vi "Meas Result Fill Freq Selector.vi"(2 "meas":T1={"swp cfg"={"N"=0, "R"=0, "f list"=[], "smpl delay"=0.0, "set delay"=0.0, "set delay np"=0.0, "meas root"=path "", "meas name"="", "meas a-index"=FALSE, "rnd sweep"=FALSE, "mode"=enum."Frequency", "swp mode"=enum."Linear", "avg"=0, "subrec"=0, "multi-freq"=FALSE, "selfcal"=FALSE, "selfcal period [h]"=0.0}, "bridge"={"type"=enum."TWM client", "TWM"={"pipe name"="", "parameters"=[], "handle"=0, "fixed aper [s]"=0.0, "f-list [Hz]"=[], "discrete f-list"=FALSE, "unc mode"=enum."None", "unc mcc"=0, "unc first"=FALSE, "alg id"=enum."TWM-LowZ - Low Z measurement"}, "last f"=0.0, "bias comp"={"bias type"=enum."dummy", "VISA"="", "Enable"=FALSE, "channel qu"=[], "channel Uinit"=[]}, "sim mode"=enum."Generic RLC network", "channel idns"=[], "sim phases"=1}, "src"={"type"=enum."Tektronix AFG3101C", "idn"="", "afg"={"VISA"="", "const"=0.0, "gen DC"=FALSE, "ext ref"=FALSE}, "cDAQ dds"={"device"="", "channels"=[], "mclk source"="", "mclk [Hz]"=0.0, "fs [Hz]"=0.0, "block [s]"=0.0, "buf [s]"=0.0, "task"="", "cmd queue"=refnum, "proc ref"=refnum, "smpl clock out"="/cDAQ3/PFI0", "export smpl clock"=FALSE, "DC ofs [V]"=[], "timebase source"="", "timebase mode"=enum."Local", "dither"=enum."Disabled", "dither level"=0.0, "phase [rad]"=[]}, "gain [V/A]"=1.0, "F5xxx session"={"VISA"="", "mode"=enum."AC voltage", "Earth on"=FALSE, "Ext ref lock"=FALSE}, "t3awg"={"VISA"="", "use ext ref"=FALSE, "ext ref [Hz]"=0.0, "load Z"=enum."High Z", "ramdac max n"=0, "noise dither [V]"=0.0, "t3awg fs rules"=[], "channels"=0, "ramdac min n"=0, "channel list"=[], "gen resl [Vpp]"=0.0, "wave data format"=enum."Binary"}}, "results"=refnum, "dvm"={"type"=enum."Disabled", "idn"="", "F5790"={"VISA"="", "Input"=enum."input 1", "Digital filter restart"=enum."medium", "hi resolution"=enum."off", "Digital filter mode"=enum."off", "ext guard"=FALSE}, "HP3458A"={"VISA"="", "ac method"=0, "resolution"=enum."6.5", "function"=0, "frequency source"=3, "auto range"=1, "manual range"=1.0}}, "thermo"={"type"=enum."COMET Tx5xx (ethernet)", "comment"="", "tag"="", "refresh"=5.0, "IP"="", "port"=502, "VISA"="", "last readout"=timestamp(0 s since 1904-01-01), "TCP ref"=refnum, "VISA sess"="", "idn"="", "press"=0.0, "RH"=0.0, "temp"=0.0, "pres cor"=[], "RH cor"=[], "temp cor"=[], "try left"=0, "failed"=FALSE, "RTD set"=[], "RTD inv"=[], "range"=0.0, "net mode"=enum."MODBUS", "try fail"=enum."Stop trying - return NaN", "timeout [s]"=0.0, "max retries"=0, "sim t [deg]"=0.0, "status"=0}} {"thermo"."status" items=["ok", "retry", "failed"]; "thermo"."RTD inv" format="%.1f"; "thermo"."RTD set" format="%.1f"; "thermo"."temp cor" format="%.1f"; "thermo"."RH cor" format="%.1f"; "thermo"."pres cor" format="%.1f"; "thermo"."refresh" min=0.1 max=1000.0 format="%.2f"; "dvm"."HP3458A"."manual range" format="%_3g"; "dvm"."HP3458A"."auto range" items=["OFF", "ON", "ONCE"]; "dvm"."HP3458A"."frequency source" items=["AC + DC Current", "AC + DC Voltage", "AC Current", "AC Voltage"]; "dvm"."HP3458A"."function" items=["DC Voltage", "AC Voltage", "AC + DC Voltage", "DC Current", "AC Current", "AC + DC Current", "2-Wire Resistance", "4-Wire Resistance", "Frequency", "Period", "Direct Sampling DC", "Direct Sampling AC", "Sub-Sampling DC", "Sub-Sampling AC"]; "dvm"."HP3458A"."ac method" items=["Analog", "Random", "Synchronous"]; "src"."t3awg"."t3awg fs rules"."fs-step [Hz]" format="%#_6p"; "src"."t3awg"."t3awg fs rules"."fs-max [Hz]" format="%#_6p"; "src"."t3awg"."t3awg fs rules"."for f0 <" format="%#_6p"; "src"."t3awg"."t3awg fs rules"."fs-min [Hz]" format="%#_6p"; "src"."cDAQ dds"."channels" min=0 step=1; "bridge"."TWM"."f-list [Hz]" format="%#_6p"; "swp cfg"."f list"."bias" format="%#_3p"; "swp cfg"."f list"."level" format="%#_3p"; "swp cfg"."f list"."fs [Hz]" format="%#_5p"; "swp cfg"."f list"."time [s]" format="%#_3p"; "swp cfg"."f list"."f/fs" format="%#_3p"; "swp cfg"."f list"."periods" format="%#_3f"; "swp cfg"."f list"."f [Hz]" format="%#_5p"}, 3 "results data":T36, 4 "res fid":refnum<vi>) -> (0 "freq filter (NaN: no filter)":dbl, 1 "freq index (default: 0)":u16)   [LabVIEW 2020]
doc: "Fills list of frequencies selector based on available sweep spots cout available in result data."
uses:
  Meas Results.ctl
  bridge/Bridge Frequency Readings Data.ctl
  drivers/TWM client/Meas Proc QWTB Spectrum Data.ctl
  drivers/TWM client/TWM Phase Info.ctl
  meas session.ctl
  Meas Sweep Config.ctl
  Meas Freq Info.ctl
  meas_swp_mode.ctl
  meas_sweep_flist_mode.ctl
  bridge/Bridge Session.ctl
  bridge/Bridge Type.ctl
  drivers/TWM client/TWM Session.ctl
  drivers/TWM client/TWM parameters.ctl
  drivers/TWM client/Meas Proc QWTB Uncertainty Mode.ctl
  bridge/Bridge Algorithm.ctl
  bridge/Bridge Bias Session.ctl
  bridge/Bridge Bias Type.ctl
  bridge/Bridge Sim Mode.ctl
  source/Source Session.ctl
  source/Source Type.ctl
  drivers/AFG3101C/AFG3101C Session.ctl
  drivers/cDAQ DDS/cDAQ DDS Session.ctl
  drivers/cDAQ DDS/cDAQ DDS Setup.ctl
  drivers/cDAQ DDS/cDAQ DDS Timebase Mode.ctl
  drivers/cDAQ DDS/cDAQ DDS Dither.ctl
  drivers/Fluke 5XXX/top_lev/F5xxx_session.ctl
  drivers/Fluke 5XXX/top_lev/F5xxx_output_mode.ctl
  drivers/T3AWG3K/toplevel/T3AWG Session.ctl
  drivers/T3AWG3K/toplevel/T3AWG Load Z.ctl
  drivers/T3AWG3K/toplevel/fgen_ramdac_fs_rules.ctl
  drivers/T3AWG3K/toplevel/T3AWG Channel.ctl
  Meas Results Ref.ctl
  dvm/dvm session.ctl
  dvm/dvm type.ctl
  drivers/Fluke 5790A/top_level/F5790 session.ctl
  drivers/Agilent 3458A/top level/HP3458A Session.ctl
  thermo/thermo.ctl
  thermo/thermo_types.ctl
  thermo/Thermometer Fail Action.ctl
  drivers/T3AWG3K/Active Technologies AWG3000.lvlib
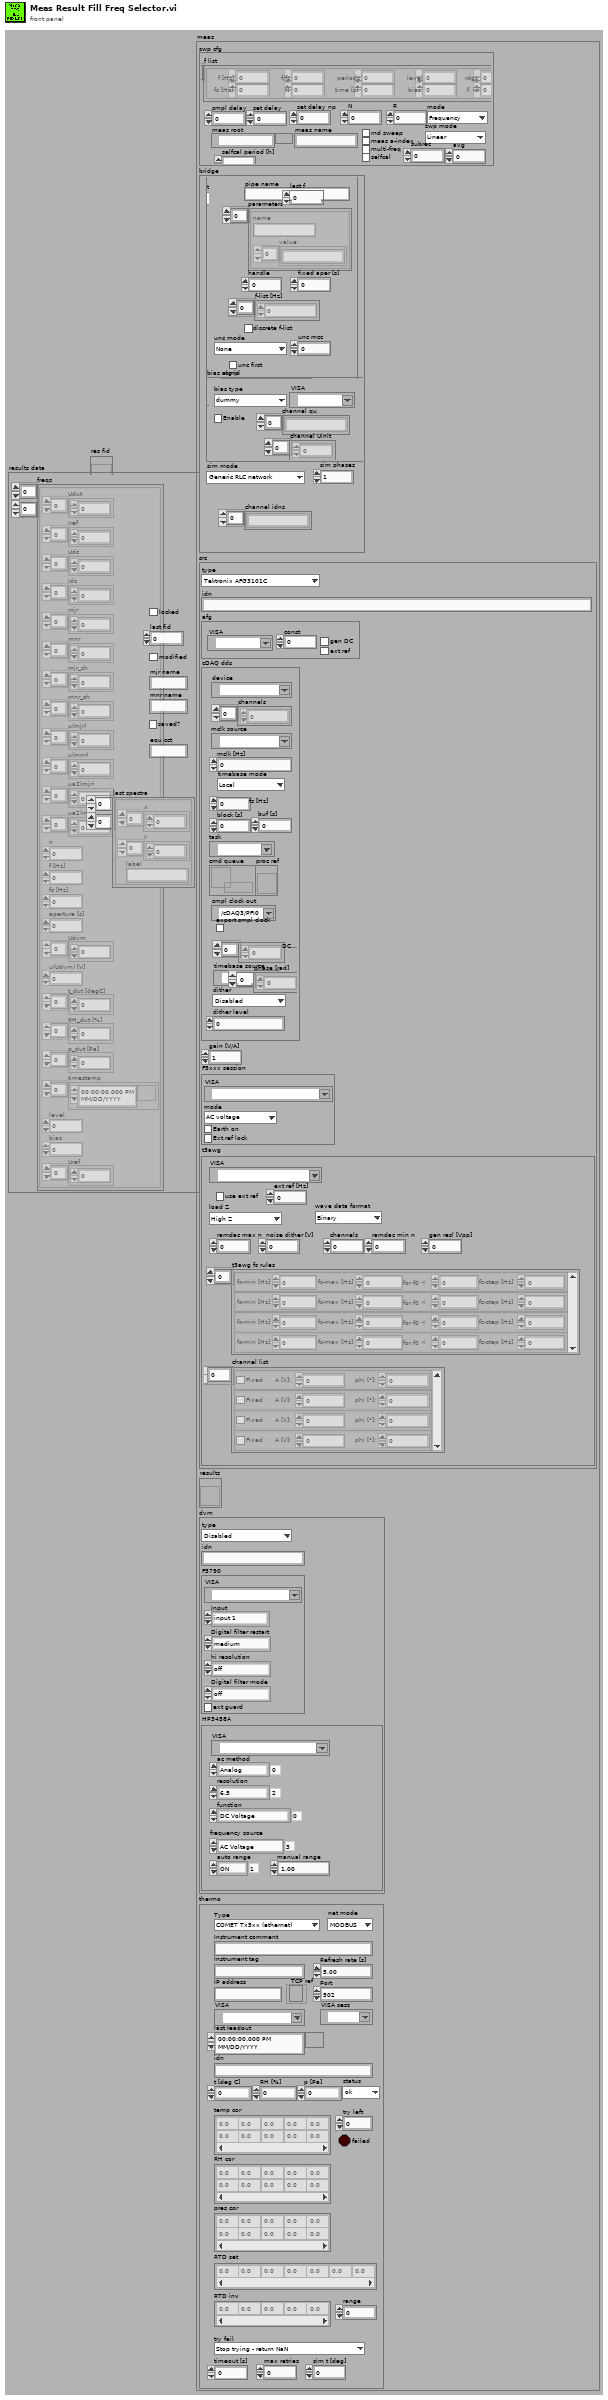
[diagram p1: front panel]
types:
  T1 = typedef "meas session.ctl" = cluster{"swp cfg":T2, "bridge":T6, "src":T15, "results":T28, "dvm":T29, "thermo":T33}
  T2 = typedef "Meas Sweep Config.ctl" = cluster{"N":i32, "R":i32, "f list":T3[], "smpl delay":dbl, "set delay":dbl, "set delay np":dbl, "meas root":path, "meas name":string, "meas a-index":bool, "rnd sweep":bool, "mode":T4, "swp mode":T5, "avg":i32, "subrec":i32, "multi-freq":bool, "selfcal":bool, "selfcal period [h]":dbl}
  T3 = typedef "Meas Freq Info.ctl" = cluster{"f [Hz]":dbl, "periods":dbl, "f/fs":dbl, "time [s]":dbl, "fs [Hz]":dbl, "N":i32, "level":dbl, "bias":dbl, "rdgs":i32, "f. id":i32}
  T4 = typedef "meas_swp_mode.ctl" = enum16{"Frequency", "Level", "Bias"}
  T5 = typedef "meas_sweep_flist_mode.ctl" = enum16{"Linear", "Log10"}
  T6 = typedef "Bridge Session.ctl" = cluster{"type":T7, "TWM":T8, "last f":dbl, "bias comp":T12, "sim mode":T14, "channel idns":string[], "sim phases":i32}
  T7 = typedef "Bridge Type.ctl" = enum16{"TWM client", "dummy"}
  T8 = typedef "TWM Session.ctl" = cluster{"pipe name":string, "parameters":T9[], "handle":i32, "fixed aper [s]":dbl, "f-list [Hz]":dbl[], "discrete f-list":bool, "unc mode":T10, "unc mcc":i32, "unc first":bool, "alg id":T11}
  T9 = typedef "TWM parameters.ctl" = cluster{"name":string, "value":string[]}
  T10 = typedef "Meas Proc QWTB Uncertainty Mode.ctl" = enum16{"None", "GUF", "Monte Carlo"}
  T11 = typedef "Bridge Algorithm.ctl" = enum16{"TWM-LowZ - Low Z measurement", "TWM-InpZ - Digitizer input Z measurement", "TWM-TIAZ - High Z using TIA"}
  T12 = typedef "Bridge Bias Session.ctl" = cluster{"bias type":T13, "VISA":refnum<visa-resource-name>, "Enable":bool, "channel qu":string[], "channel Uinit":dbl[]}
  T13 = typedef "Bridge Bias Type.ctl" = enum16{"dummy", "CMI LiBbias V1.0"}
  T14 = typedef "Bridge Sim Mode.ctl" = enum16{"Generic RLC network", "Interchannel transfer", "Input impedance"}
  T15 = typedef "Source Session.ctl" = cluster{"type":T16, "idn":string, "afg":T17, "cDAQ dds":T18, "gain [V/A]":dbl, "F5xxx session":T21, "t3awg":T23}
  T16 = typedef "Source Type.ctl" = enum16{"Tektronix AFG3101C", "cDAQ DAC", "Fluke 5xxx", "Datron 4xxx", "Agilent 33120A", "R&S SMT", "Teledyne LeCroy T3AWG", "dummy"}
  T17 = typedef "AFG3101C Session.ctl" = cluster{"VISA":refnum<visa-resource-name>, "const":dbl, "gen DC":bool, "ext ref":bool}
  T18 = typedef "cDAQ DDS Session.ctl" = cluster{"device":tag, "channels":i32[], "mclk source":tag, "mclk [Hz]":dbl, "fs [Hz]":dbl, "block [s]":dbl, "buf [s]":dbl, "task":refnum<k21>, "cmd queue":refnum<queue>, "proc ref":refnum<vi>, "smpl clock out":tag, "export smpl clock":bool, "DC ofs [V]":dbl[], "timebase source":tag, "timebase mode":T19, "dither":T20, "dither level":dbl, "phase [rad]":dbl[]}
  T19 = typedef "cDAQ DDS Timebase Mode.ctl" = enum16{"Local", "Take from ADC (e.g. NI 9238)", "Other source"}
  T20 = typedef "cDAQ DDS Dither.ctl" = enum16{"Disabled", "Gaussian"}
  T21 = typedef "F5xxx_session.ctl" = cluster{"VISA":refnum<visa-resource-name>, "mode":T22, "Earth on":bool, "Ext ref lock":bool}
  T22 = typedef "F5xxx_output_mode.ctl" = enum16{"AC voltage", "AC current"}
  T23 = typedef "Active Technologies AWG3000.lvlib/T3AWG Session.ctl" = cluster{"VISA":refnum<visa-resource-name>, "use ext ref":bool, "ext ref [Hz]":dbl, "load Z":T24, "ramdac max n":i32, "noise dither [V]":dbl, "t3awg fs rules":T25[], "channels":i32, "ramdac min n":i32, "channel list":T26[], "gen resl [Vpp]":dbl, "wave data format":T27}
  T24 = typedef "Active Technologies AWG3000.lvlib/T3AWG Load Z.ctl" = enum16{"High Z", "50 Ohm"}
  T25 = typedef "Active Technologies AWG3000.lvlib/fgen_ramdac_fs_rules.ctl" = cluster{"fs-min [Hz]":dbl, "fs-max [Hz]":dbl, "for f0 < ":dbl, "fs-step [Hz]":dbl}
  T26 = typedef "Active Technologies AWG3000.lvlib/T3AWG Channel.ctl" = cluster{"Fixed":bool, "A [V]:":dbl, "phi [°]:":dbl}
  T27 = typedef "Active Technologies AWG3000.lvlib/T3AWG Wave Format" = enum16{"Text", "Binary"}
  T28 = typedef "Meas Results Ref.ctl" = refnum<vi>
  T29 = typedef "dvm session.ctl" = cluster{"type":T30, "idn":string, "F5790":T31, "HP3458A":T32}
  T30 = typedef "dvm type.ctl" = enum16{"Disabled", "Simulated", "Fluke 5790A", "Keysight 3458A"}
  T31 = typedef "F5790 session.ctl" = cluster{"VISA":refnum<visa-resource-name>, "Input":enum16{"input 1", "input 2", "wide-band"}, "Digital filter restart":enum16{"medium", "fine", "coarse"}, "hi resolution":enum16{"off", "on"}, "Digital filter mode":enum16{"off", "fast", "medium", "slow"}, "ext guard":bool}
  T32 = typedef "HP3458A Session.ctl" = cluster{"VISA":refnum<visa-resource-name>, "ac method":u16, "resolution":enum16{"4.5", "5.5", "6.5", "7.5", "8.5"}, "function":u16, "frequency source":u16, "auto range":u16, "manual range":dbl}
  T33 = typedef "thermo.ctl" = cluster{"type":T34, "comment":string, "tag":string, "refresh":dbl, "IP":string, "port":u16, "VISA":refnum<visa-resource-name>, "last readout":timestamp, "TCP ref":refnum<k5>, "VISA sess":refnum<visa-resource-name>, "idn":string, "press":dbl, "RH":dbl, "temp":dbl, "pres cor":dbl[][], "RH cor":dbl[][], "temp cor":dbl[][], "try left":i32, "failed":bool, "RTD set":dbl[], "RTD inv":dbl[], "range":dbl, "net mode":enum16{"MODBUS", "HTTP"}, "try fail":T35, "timeout [s]":dbl, "max retries":i32, "sim t [deg]":dbl, "status":u16}
  T34 = typedef "thermo_types.ctl" = enum16{"Disabled", "Simulated", "COMET Tx5xx (ethernet)", "Keithley 2002 (GPIB) + RTD", "Agilent 344xx (GPIB) + RTD"}
  T35 = typedef "Thermometer Fail Action.ctl" = enum16{"Stop trying - keep last value", "Stop trying - return NaN", "Generate error - stop sweep"}
  T36 = typedef "Meas Results.ctl" = cluster{"freqs":T37[][], "locked":bool, "last fid":i32, "modified":bool, "mjr name":string, "mnr name":string, "last spectra":T38[][], "saved?":bool, "TWM phase":T39[], "time start":timestamp, "time stop":timestamp, "equ cct":string}
  T37 = typedef "Bridge Frequency Readings Data.ctl" = cluster{"Udut":dbl[], "Iref":dbl[], "Udc":dbl[], "Idc":dbl[], "mjr":dbl[], "mnr":dbl[], "mjr_sh":dbl[], "mnr_sh":dbl[], "u(mjr)":dbl[], "u(mnr)":dbl[], "ua2(mjr)":dbl[], "ua2(mnr)":dbl[], "n":i32, "f [Hz]":dbl, "fs [Hz]":dbl, "aperture [s]":dbl, "Udvm":dbl[], "u(Udvm) [V]":dbl, "t_dut [degC]":dbl[], "RH_dut [%]":dbl[], "p_dut [Pa]":dbl[], "timestamp":timestamp[], "level":dbl, "bias":dbl, "Uref":dbl[]}
  T38 = typedef "Meas Proc QWTB Spectrum Data.ctl" = cluster{"x":sgl[], "y":sgl[], "label":string}
  T39 = typedef "TWM Phase Info.ctl" = cluster{"ref chn id (I)":string, "dut chn id (U)":string, "ref chn range [V]":dbl, "dut chn range [V]":dbl, "aperture [s]":dbl, "fs [Hz]":dbl, "ref chn transducer (I)":string, "dut chn transducer (U)":string}
  T40 = enum8{"Enabled", "Disabled", "Disabled and Grayed Out"}
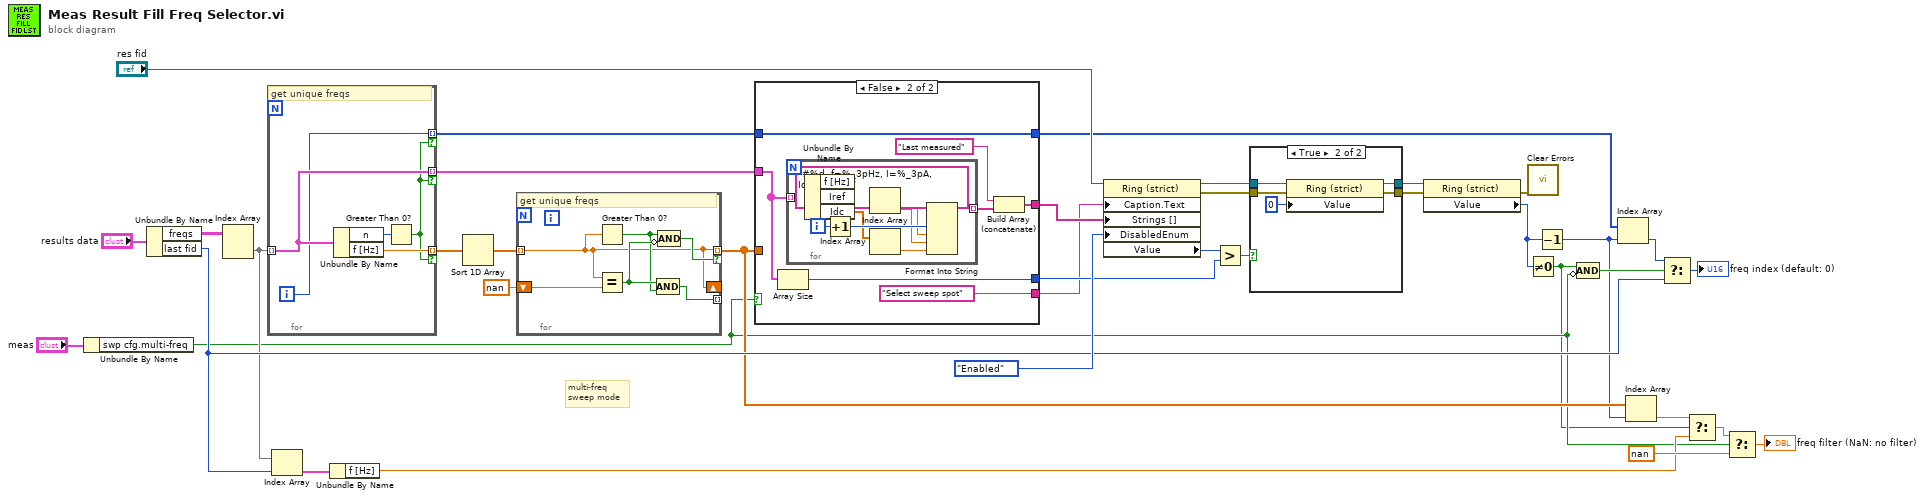
[diagram p0: block diagram]
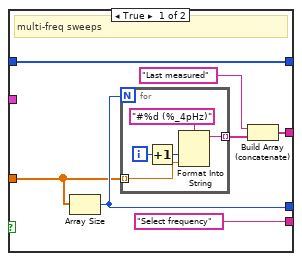
[diagram p2: hidden frame]
diagram:
  # "multi-freq\nsweep mode"
  n1 = Unbundle By Name("meas") -> ("swp cfg.multi-freq"=w10:bool)
  n2 = Unbundle By Name("results data") -> ("freqs"=w32:T37[][], "last fid"=w22:i32)
  n3 = Index Array(array=w32) -> (element=w20:T37[])  [unwired: 2 in]
  n4 = for {
    tunnel: w20 -> [w40] mode=indexing
    tunnel: [w42] -> w15 mode=indexing if=w38
    tunnel: [w40] -> w5 mode=indexing if=w38
    tunnel: [w39] -> w4 mode=indexing if=w38
    i -> [w39]
    # "get unique freqs"
    n5 = Unbundle By Name(w40) -> ("n"=w41:i32, "f [Hz]"=w42:dbl)
    n6 = Greater Than 0?(x=w41) -> (x > 0?=w38:bool)
  }
  n7 = Index Array(array=w20, index=w22) -> (element=w21:T37)
  n8 = Unbundle By Name(w21) -> ("f [Hz]"=w18:dbl)
  n9 = Sort 1D Array(array=w15) -> (sorted array=w12:dbl[])
  n10 = for {
    tunnel: w12 -> [w43] mode=indexing
    shift-right: [w43] -> _
    shift-left: nan ("f [Hz]") -> [w48]
    tunnel: [w44] -> _ mode=indexing
    tunnel: [w43] -> w13 mode=indexing if=w47
    # "get unique freqs"
    n11 = Greater Than 0?(x=w43) -> (x > 0?=w45:bool)
    n12 = Equal?(x=w43, y=w48) -> (x = y?=w46:bool)
    n13 = Compound Arithmetic op=AND(w46, w45) -> (w44:bool)
    n14 = Compound Arithmetic op=AND(w45, invert w46) -> (w47:bool)
  }
  n15 = case shown="False" w10 {
    tunnel: [w55 w67] -> w26
    tunnel: w13 -> [w54 _]
    tunnel: [w53 w66] -> w25
    tunnel: w5 -> [_ w61]
    tunnel: ["Select frequency" "Select sweep spot"] -> w17
    tunnel: w4 -> [w49 w62]
    tunnel: [w49 w62] -> w2
    frame True {
      # "multi-freq sweeps"
      n16 = Array Size(array=w54) -> (size(s)=w55:i32)
      n17 = for {
        N: w55 -> [_]
        tunnel: [w57] -> w52 mode=indexing
        tunnel: w54 -> [w56] mode=indexing
        i -> [w60]
        n18 = Increment(x=w60) -> (x+1=w59:i32)
        n19 = Format Into String(format string="#%d (%_4pHz)", w59, w56) -> (resulting string=w57:string)  [unwired: 2 in, 1 out]
      }
      n20 = Build Array (concatenate)("Last measured", w52) -> (w53:string[])
    }
    frame False {
      n21 = Array Size(array=w61) -> (size(s)=w67:i32)
      n22 = for {
        tunnel: [w74] -> w65 mode=indexing
        tunnel: w61 -> [w73] mode=indexing
        i -> [w77]
        n23 = Unbundle By Name(w73) -> ("f [Hz]"=w72:dbl, "Iref"=w71:dbl[], "Idc"=w69:dbl[])
        n24 = Increment(x=w77) -> (x+1=w76:i32)
        n25 = Index Array(array=w71) -> (element=w70:dbl)  [unwired: 1 in]
        n26 = Index Array(array=w69) -> (element=w68:dbl)  [unwired: 1 in]
        n27 = Format Into String(format string="#%d, f=%_3pHz, I=%_3pA, Idc=%_3pA", w76, w72, w70, w68) -> (resulting string=w74:string)  [unwired: 2 in, 1 out]
      }
      n28 = Build Array (concatenate)("Last measured", w65) -> (w66:string[])
    }
  }
  n29 = property class="Ring (strict)"(reference="res fid", "Caption.Text"=w17, "Strings []"=w25, "DisabledEnum"=T40."Enabled" ("Disabled")) -> (reference out=w27:refnum<vi>, error out=w28:errorcluster, "Value"=w30:u16)  [unwired: 1 in]
  n30 = Greater?(x=w30, y=w26) -> (0:w29:bool)
  n31 = case shown="True" w29 {
    tunnel: w28 -> [w79 w84]
    tunnel: w27 -> [w78 w83]
    tunnel: [w79 w81] -> w35
    tunnel: [w78 w80] -> w34
    frame False {
    }
    frame True {
      n32 = property class="Ring (strict)"(reference=w83, error in=w84, "Value"=u16 0) -> (reference out=w80:refnum<vi>, error out=w81:errorcluster)
    }
  }
  n33 = property class="Ring (strict)"(reference=w34, error in=w35) -> (error out=w33:errorcluster, "Value"=w23:u16)  [unwired: 1 out]
  n34 = call <vilib>:"Clear Errors.vi"("error in (no error)"=w33) -> ()  [unwired: 5 in, 2 out]
  n35 = Not Equal To 0?(x=w23) -> (x != 0?=w9:bool)
  n36 = Decrement(x=w23) -> (x-1=w1:u16)
  n37 = Compound Arithmetic op=AND(w9, invert w10) -> (w11:bool)
  n38 = Index Array(array=w2, index=w1) -> (element=w3:i32)
  n39 = Index Array(array=w13, index=w1) -> (element=w7:dbl)
  n40 = Select(t=w3, s=w11, f=w22) -> (s? t:f=→"freq index (default: 0)":i32)
  n41 = Select(t=w7, s=w9, f=w18) -> (s? t:f=w6:dbl)
  n42 = Select(t=w6, s=w10, f=nan) -> (s? t:f=→"freq filter (NaN: no filter)":dbl)
